vi "Create Shared Resources.vi"(8 "error in":errorcluster, 10 "custom device ref":T1=18446744073709551615 format="%.0x", 11 "Shared Resources Factory in":refnum<class "Shared Resources Factory.lvclass">) -> (0 "error out":errorcluster, 2 "shared resources":refnum<class "Shared Resources.lvclass">, 3 "Shared Resources Factory out":refnum<class "Shared Resources Factory.lvclass">)   [LabVIEW 2020, in "Ballard MIL-STD-1553 Engine.lvlib" / "Implementation.lvlib" / "Shared Resources Factory.lvclass"]
uses:
  Shared Resources Factory.lvclass
  <vilib>/NI VeriStand/Custom Device API/Custom Device Item Ref.ctl
  Interfaces/Shared Resources/Shared Resources.lvclass
  Shared Resources/Shared Resources.lvclass
  Shared/Initialization Method.ctl
  Shared/Device Parameters.ctl
  C:/dev/niveristand-ballard-milStd1553-custom-device/Source/Custom Device Support/Engine/Implementation/Shared Resources/Shared Resources.lvclass
  C:/dev/niveristand-ballard-milStd1553-custom-device/Source/Custom Device Support/Engine/Interfaces/Shared Resources/Shared Resources.lvclass
  <vilib>/NI VeriStand/Custom Device API/Custom Device API.lvlib
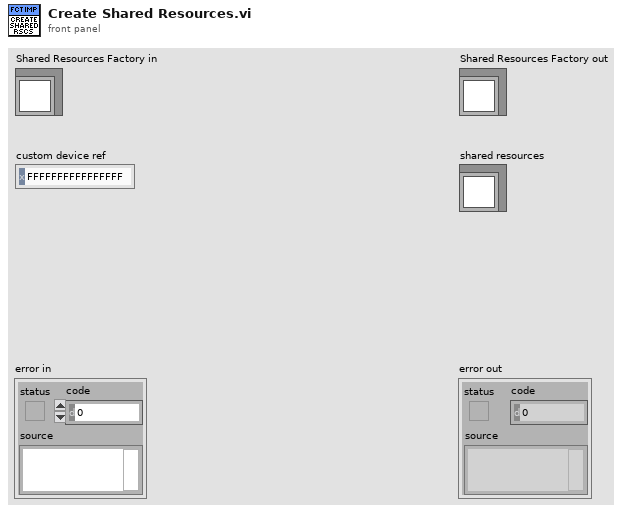
[diagram p1: front panel]
types:
  T1 = typedef "Custom Device API.lvlib/Custom Device Item Ref.ctl" = u64
  T2 = typedef "Device Parameters.ctl" = cluster{"initialization method":T3, "card number":i32, "PXI slot number":i32, "core number":i32}
  T3 = typedef "Initialization Method.ctl" = enum16{"PXI Slot Number", "Card Number"}
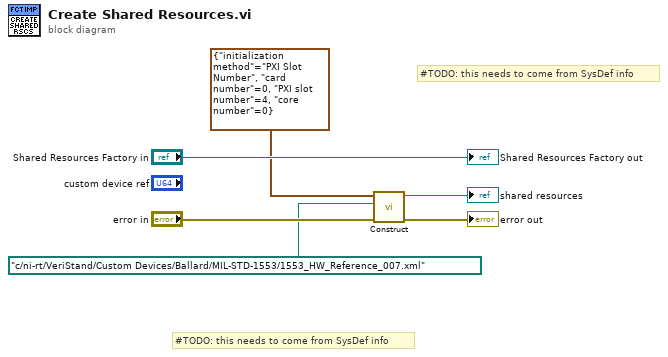
[diagram p0: block diagram]
diagram:
  # "#TODO: this needs to come from SysDef info"
  # "#TODO: this needs to come from SysDef info"
  n1 = call "Construct.vi"("error in (no error)"="error in", "hardware config file"=path "c:/ni-rt/VeriStand/Custom Devices/Ballard/MIL-STD-1553/1553_HW_Reference_007.xml", "device parameters"=T2 {"initialization method"=enum."PXI Slot Number", "card number"=0, "PXI slot number"=4, "core number"=0}) -> ("error out"=→"error out":errorcluster, "Ballard 1553 shared resources"=→"shared resources":refnum<class "Shared Resources.lvclass">)  [unwired: 7 in]
  "Shared Resources Factory out" <- "Shared Resources Factory in"
